vi "__uintLCM.vi"(8 "Base (decimal)":T1=10 items=["Binary"=2, "Octal"=8, "Decimal"=10, "Hexadecimal"=16, "Hexatrigesimal"=36, "ASCII"=64], 10 "Uint2 in":u8[](array[numeric])=[0], 11 "Uint1 in":u8[](array[numeric])=[0]) -> (0 "Timing":u32, 3 "LCM(Int1,Int2)":u8[](array[numeric]))   [LabVIEW 2011, in "UintClass.lvclass"]
uses:
  UintClass.lvclass
  enumBase.ctl
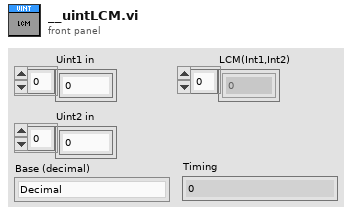
[diagram p1: front panel]
types:
  T1 = typedef "UintClass.lvclass/enumBase.ctl" = u16
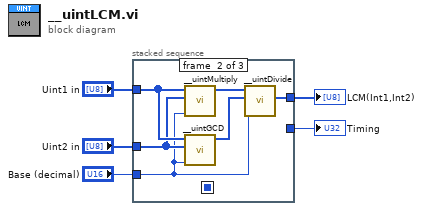
[diagram p0: block diagram]
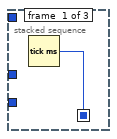
[diagram p2: hidden frame]
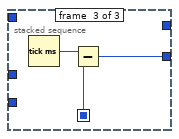
[diagram p3: hidden frame]
diagram:
  n1 = stacked-sequence {
    seq-local: [w6 _ _] -> [_ _ w14]
    tunnel: "Uint1 in" -> [_ w12 _]
    tunnel: "Uint2 in" -> [_ w10 _]
    tunnel: "Base (decimal)" -> [_ w8 _]
    tunnel: [_ w7 _] -> w2
    tunnel: [_ _ w13] -> w1
    frame #0 {
      n2 = Tick Count (ms)() -> (millisecond timer value=w6:u32)
    }
    frame #1 {
      n3 = call "__uintMultiply.vi"("Base (decimal)"=w8, "UInt2 in"=w10, "UInt1 in"=w12) -> ("UInt1 * Uint2"=w11:u8[])  [unwired: 7 in, 1 out]
      n4 = call "__uintGCD.vi"("Base (decimal)"=w8, "Uint2 in"=w10, "Uint1 in"=w12) -> ("GCD(Int1,Int2)"=w9:u8[])  [unwired: 7 in, 1 out]
      n5 = call "__uintDivide.vi"("Base (decimal)"=w8, "Uint2 in"=w9, "Uint1 in"=w11) -> ("floor(Uint1 / Uint1)"=w7:u8[])  [unwired: 6 in, 2 out]
    }
    frame #2 {
      n6 = Tick Count (ms)() -> (millisecond timer value=w15:u32)
      n7 = Subtract(x=w15, y=w14) -> (x-y=w13:u32)
    }
  }
  "LCM(Int1,Int2)" <- w2
  "Timing" <- w1
